vi "Test Target has one Additional Char.vi"(11 "Test Case In":refnum<class "Added Section Finder Test.lvclass">) -> (0 "error out":errorcluster, 3 "Test Case Out":refnum<class "Added Section Finder Test.lvclass">)   [LabVIEW 2020, in "Added Section Finder Test.lvclass"]
uses:
  Added Section Finder Test.lvclass
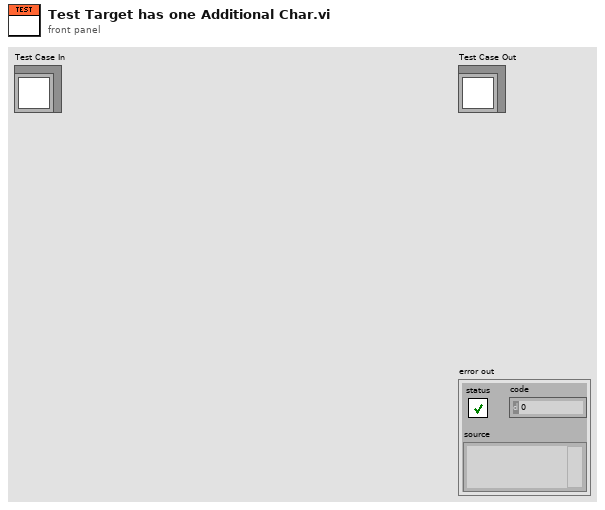
[diagram p1: front panel]
types:
  T1 = cluster{"Selection Start":u32, "Selection End":u32}
  T2 = cluster{"Selection Start":u32, "Selection End":u32}[]
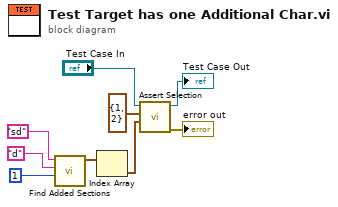
[diagram p0: block diagram]
diagram:
  n1 = call "Find Added Sections.vi"("Offset"=u32 1 ("Index"), "Reference"="d", "Target"="sd") -> ("Sections in Target"=w6:T2)  [unwired: 8 in]
  n2 = Index Array(array=w6) -> (element=w3:T1)  [unwired: 1 in]
  n3 = call "Assert Selection.vi"("Actual"=w3, "Expected"=T1 {"Selection Start"=1, "Selection End"=2} ("Text.Selection"), "Added Section Finder Test In"="Test Case In") -> ("error out"=→"error out":errorcluster, "Added Section Finder Test Out"=→"Test Case Out":refnum<class "Added Section Finder Test.lvclass">)  [unwired: 7 in]
